vi "HEWH Check Final Conditions.vi"(8 "Error In":errorcluster, 10 "Start Draw":bool, 11 "Test Complete":bool) -> (0 "Error Out":errorcluster, 3 "Prevent More Draws":bool)   [LabVIEW 2016]
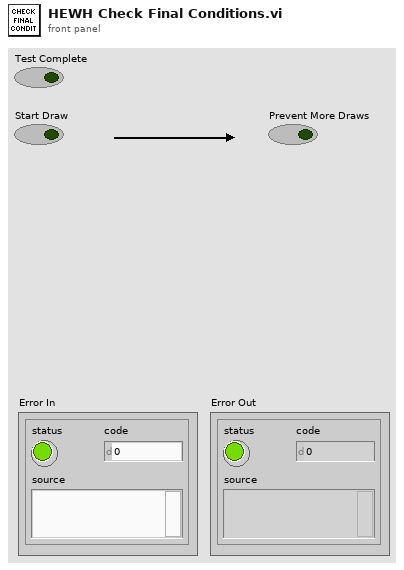
[diagram p1: front panel]
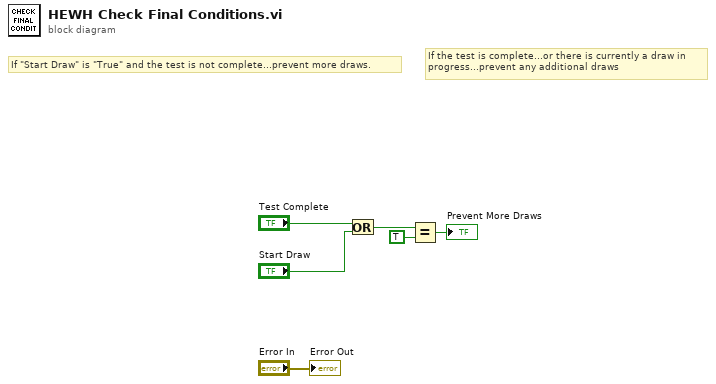
[diagram p0: block diagram]
diagram:
  # "If \"Start Draw\" is \"True\" and the test is not complete...prevent more draws."
  # "If the test is complete...or there is currently a draw in \nprogress...prevent any additional draws"
  n1 = Or(x="Test Complete", y="Start Draw") -> (x .or. y?=w6:bool)
  n2 = Equal?(x=w6, y=TRUE) -> (x = y?=→"Prevent More Draws":bool)
  "Error Out" <- "Error In"
